vi "Get_Prompt.vi"(1 "Event":cluster{string, string[], dbl[], dbl}) -> (0 "Prompt":string)   [LabVIEW 2011]
doc: "This VI determines what \"Prompt\" (string) the user has specified for a given event, returning a default prompt if none was found."
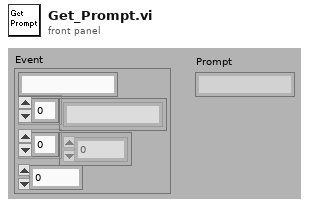
[diagram p1: front panel]
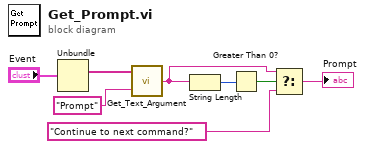
[diagram p0: block diagram]
diagram:
  n1 = Unbundle("Event") -> (w7:string[])  [unwired: 3 out]
  n2 = call "Get_Text_Argument.vi"("Argument"="Prompt", "Argument List"=w7) -> ("Text"=w3:string)
  n3 = String Length(string=w3) -> (length=w5:i32)
  n4 = Greater Than 0?(x=w5) -> (x > 0?=w4:bool)
  n5 = Select(t=w3, s=w4, f="Continue to next command?") -> (s? t:f=→"Prompt":string)
